vi "libssh2_agent_publickey_free.vi"(8 "error in (no error)":errorcluster, 11 "public key":T1) -> (0 "error out":errorcluster)   [LabVIEW 2013, in "libssh2.lvlib"]
doc: "Frees ressources associated with <B>public key</B>."
uses:
  libssh2.lvlib
  libssh2_agent_publickey_refnum.ctl
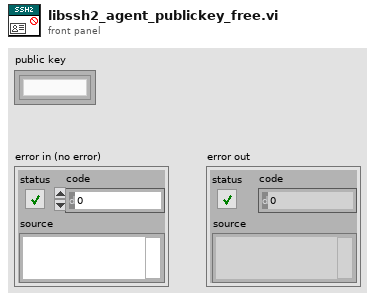
[diagram p1: front panel]
types:
  T1 = typedef "libssh2.lvlib/libssh2_agent_publickey_refnum.ctl" = refnum<k1>
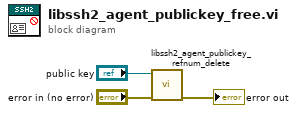
[diagram p0: block diagram]
diagram:
  n1 = call "libssh2_agent_publickey_refnum_delete.vi"("error in (no error)"="error in (no error)", "public key"="public key") -> ("error out"=→"error out":errorcluster)  [unwired: 8 in, 1 out]
